vi "滾球機.vi"() -> ()   [LabVIEW 2018]
uses:
  <vilib>/myRIO/Common/Instrument Driver Framework/Utilities/typedefs/Generic FPGA Reference.ctl
  <vilib>/myRIO/Common/Instrument Driver Framework/Utilities/typedefs/myRIO v1.0 Reference.ctl
  <vilib>/myRIO/Common/Instrument Driver Framework/Utilities/typedefs/Hardware Version Enum.ctl
  <vilib>/myRIO/Common/Instrument Driver Framework/Utilities/typedefs/myRIO Generic Hardware Reference.ctl
  <vilib>/userdefined/High Color/nirio_resource_hc.ctl
  <vilib>/myRIO/Common/Instrument Driver Framework/Utilities/vis/Is FPGA Ref Available.vi
  <vilib>/myRIO/Express VI/Onboard IO/DI/DI Express VI.xnode
  <vilib>/myRIO/Instrument Drivers/Onboard IO/DIO/vis/Read.vi
  <vilib>/myRIO/Instrument Drivers/Onboard IO/DIO/DIO.lvlib
  <vilib>/myRIO/Common/Instrument Driver Framework/myRIO v1.0/DIO/typedefs/DIO Channels Enum.ctl
  <vilib>/myRIO/Common/Instrument Driver Framework/myRIO v1.0/DIO/typedefs/DIO Channels List.ctl
  <vilib>/myRIO/Instrument Drivers/Onboard IO/DIO/typedefs/DIO Reference.ctl
  <vilib>/myRIO/Instrument Drivers/Onboard IO/DIO/vis/myRIO DIO Open.xnode
  <vilib>/myRIO/Common/Instrument Driver Framework/myRIO v1.0/DIO/vis/myRIO v1.1 Open DIO.vi
  <vilib>/myRIO/Express VI/Onboard IO/PWM/PWM Express VI.xnode
  <vilib>/myRIO/Instrument Drivers/Onboard IO/PWM/vis/Set Duty Cycle and Frequency.vi
  <vilib>/myRIO/Instrument Drivers/Onboard IO/PWM/PWM.lvlib
  <vilib>/myRIO/Instrument Drivers/Onboard IO/PWM/typedefs/PWM Configuration.ctl
  <vilib>/myRIO/Common/Instrument Driver Framework/myRIO v1.0/PWM/typedefs/PWM Channels Enum.ctl
  <vilib>/myRIO/Instrument Drivers/Onboard IO/PWM/typedefs/PWM Reference.ctl
  <vilib>/myRIO/Instrument Drivers/Onboard IO/PWM/vis/myRIO PWM Open.xnode
  <vilib>/myRIO/Common/Instrument Driver Framework/myRIO v1.0/PWM/vis/myRIO v1.1 Open PWM.vi
panel:
  out "Tab Control":enum32{"Page 1", "Page 2"}(tab)
  in  "stop":bool
  in  "難度":bool
  out "String":string
  in  "OK Button 困難(雙人)":bool
  in  "OK Button 簡單(單人)":bool
  out "Boolean 5":bool
  out "Boolean 4":bool
  out "Boolean 3":bool
  out "Boolean 2":bool
  out "Boolean":bool
  in  "stop 2":bool
  out "得分":dbl
  out "總分":dbl
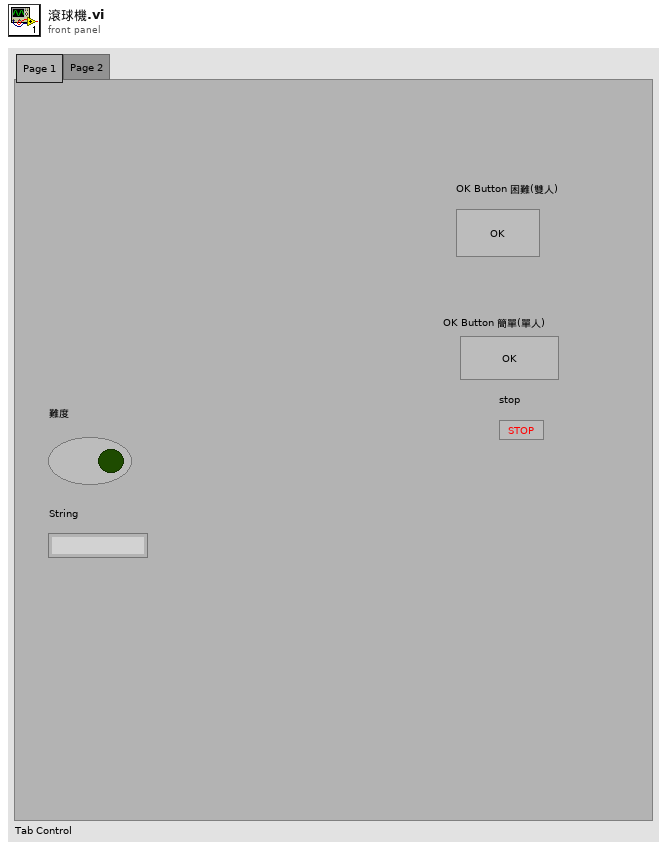
[diagram p1: front panel]
types:
  T1 = typedef "DIO.lvlib/DIO Reference.ctl" = cluster{"myRIO Reference":T2, "DIO Channels List":T6}
  T2 = typedef "myRIO Generic Hardware Reference.ctl" = cluster{"myRIO Model":T3, "myRIO Hardware Reference":T4}
  T3 = typedef "Hardware Version Enum.ctl" = enum16{"Unknown", "myRIO-1900", "myRIO-1950", "roboRIO", "NI ELVIS RIO CM", "ELVIS III"}
  T4 = typedef "myRIO v1.0 Reference.ctl" = cluster{"Generic FPGA Reference":T5, "Allow multiple opens":bool}
  T5 = typedef "Generic FPGA Reference.ctl" = refnum<k20>
  T6 = typedef "DIO Channels List.ctl" = T7[]
  T7 = typedef "DIO Channels Enum.ctl" = enum16{"Not Connected", "C/DIO0", "C/DIO1", "C/DIO2", "C/DIO3", "C/DIO4", "C/DIO5", "C/DIO6", "C/DIO7", "A/DIO0", "A/DIO1", "A/DIO2", "A/DIO3", "A/DIO4", "A/DIO5", "A/DIO6", "A/DIO7", "A/DIO8", "A/DIO9", "A/DIO10", "A/DIO11", "A/DIO12", "A/DIO13", "A/DIO14", "A/DIO15", "A/DIO16", "A/DIO17", "A/DIO18", "A/DIO19", "B/DIO0", "B/DIO1", "B/DIO2", "B/DIO3", "B/DIO4", "B/DIO5", "B/DIO6", "B/DIO7", "B/DIO8", "B/DIO9", "B/DIO10", "B/DIO11", "B/DIO12", "B/DIO13", "B/DIO14", "B/DIO15", "B/DIO16", "B/DIO17", "B/DIO18", "B/DIO19", "LED0", "LED1", "LED2", "LED3", "Button0", "DIO/DIO0", "DIO/DIO1", "DIO/DIO2", "DIO/DIO3", "DIO/DIO4", "DIO/DIO5", "DIO/DIO6", "DIO/DIO7", "DIO/DIO8", "DIO/DIO9", "SPI/CS0", "SPI/CS1", "SPI/CS2", "SPI/CS3", "LED RADIO (Green)", "LED RADIO (Red)", "LED COMM (Green)", "LED COMM (Red)", "LED MODE (Green)", "LED MODE (Red)"}
  T8 = typedef "nirio_resource_hc.ctl" = tag
  T9 = typedef "PWM.lvlib/PWM Reference.ctl" = cluster{"myRIO Reference":T2, "PWM Channels Enum":T10, "PWM Configuration":T11}
  T10 = typedef "PWM Channels Enum.ctl" = enum16{"Not Connected", "C/PWM0", "C/PWM1", "A/PWM0", "A/PWM1", "A/PWM2", "A/PWM3", "A/PWM4", "A/PWM5", "A/PWM6", "A/PWM7", "A/PWM8", "A/PWM9", "A/PWM10", "A/PWM11", "A/PWM12", "A/PWM13", "A/PWM14", "A/PWM15", "A/PWM16", "A/PWM17", "A/PWM18", "A/PWM19", "B/PWM0", "B/PWM1", "B/PWM2", "B/PWM3", "B/PWM4", "B/PWM5", "B/PWM6", "B/PWM7", "B/PWM8", "B/PWM9", "B/PWM10", "B/PWM11", "B/PWM12", "B/PWM13", "B/PWM14", "B/PWM15", "B/PWM16", "B/PWM17", "B/PWM18", "B/PWM19", "PWM/PWM0", "PWM/PWM1", "PWM/PWM2", "PWM/PWM3", "PWM/PWM4", "PWM/PWM5", "PWM/PWM6", "PWM/PWM7", "PWM/PWM8", "PWM/PWM9"}
  T11 = typedef "PWM.lvlib/PWM Configuration.ctl" = cluster{"Frequency":dbl, "Duty Cycle":dbl}
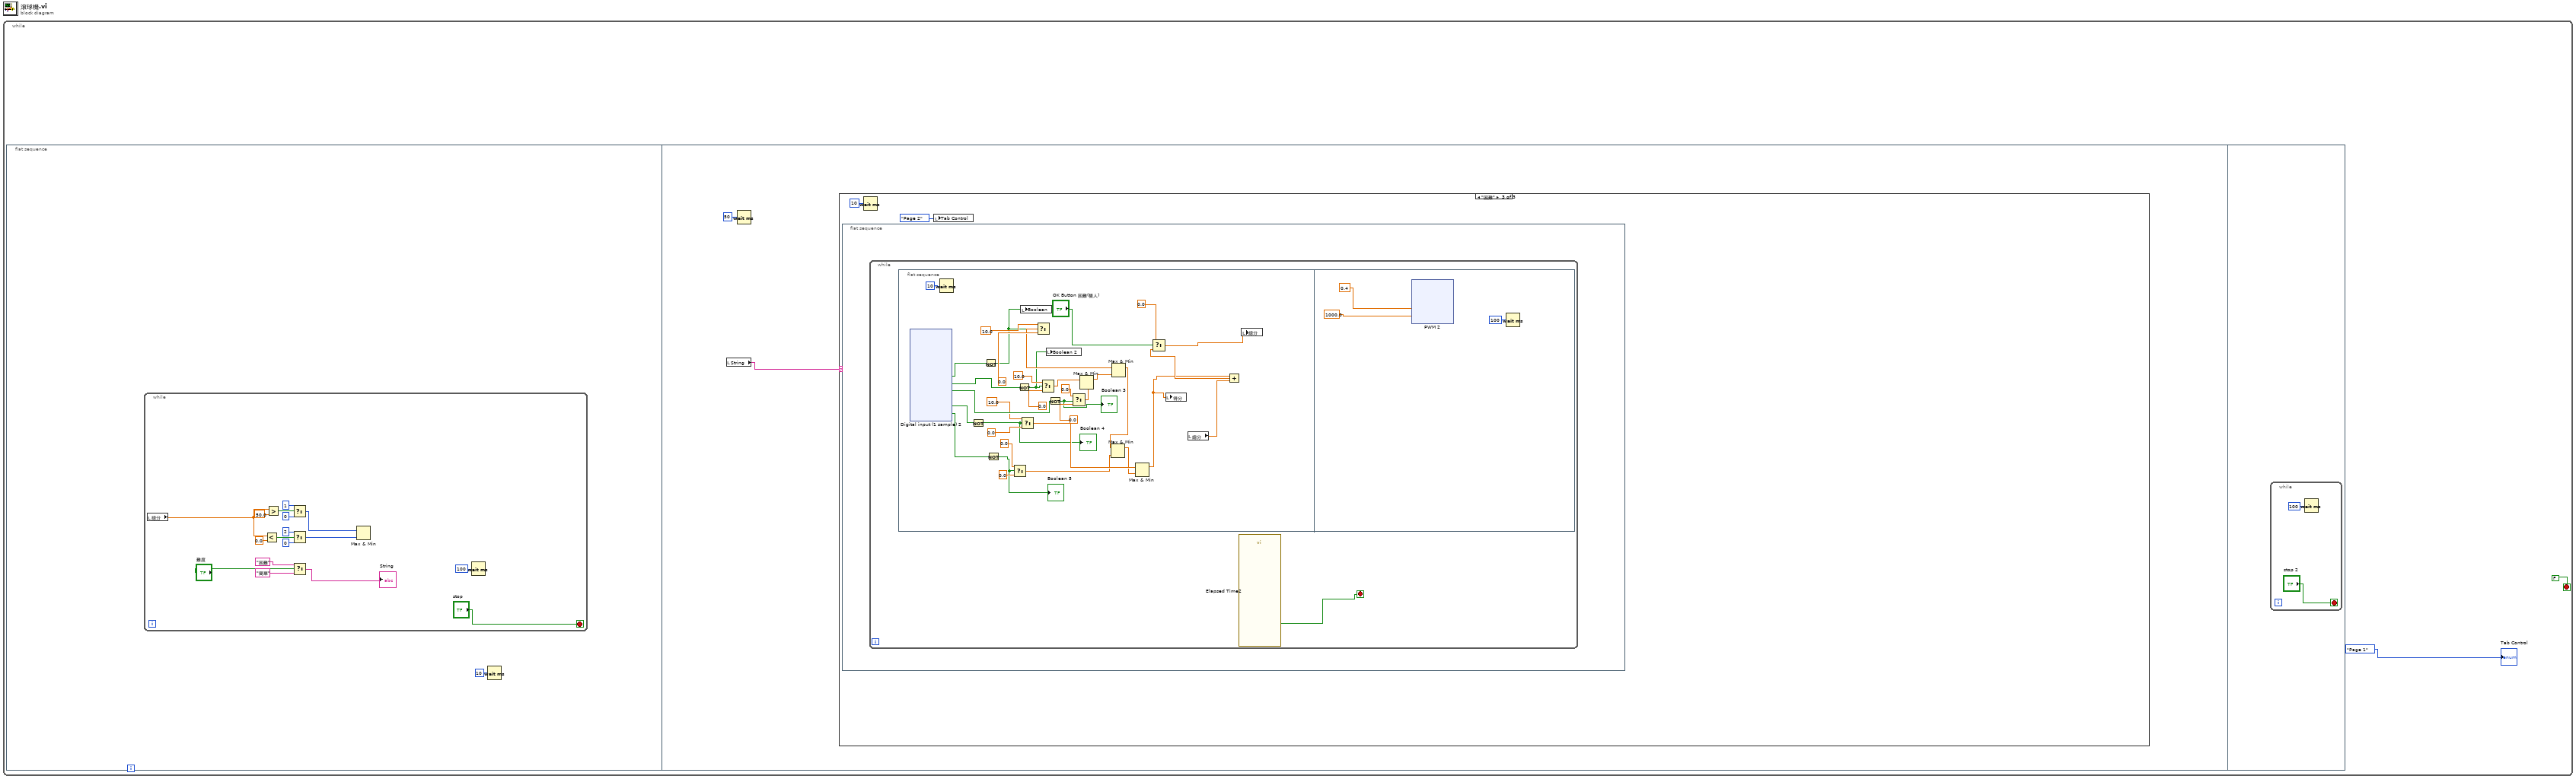
[diagram p0: block diagram]
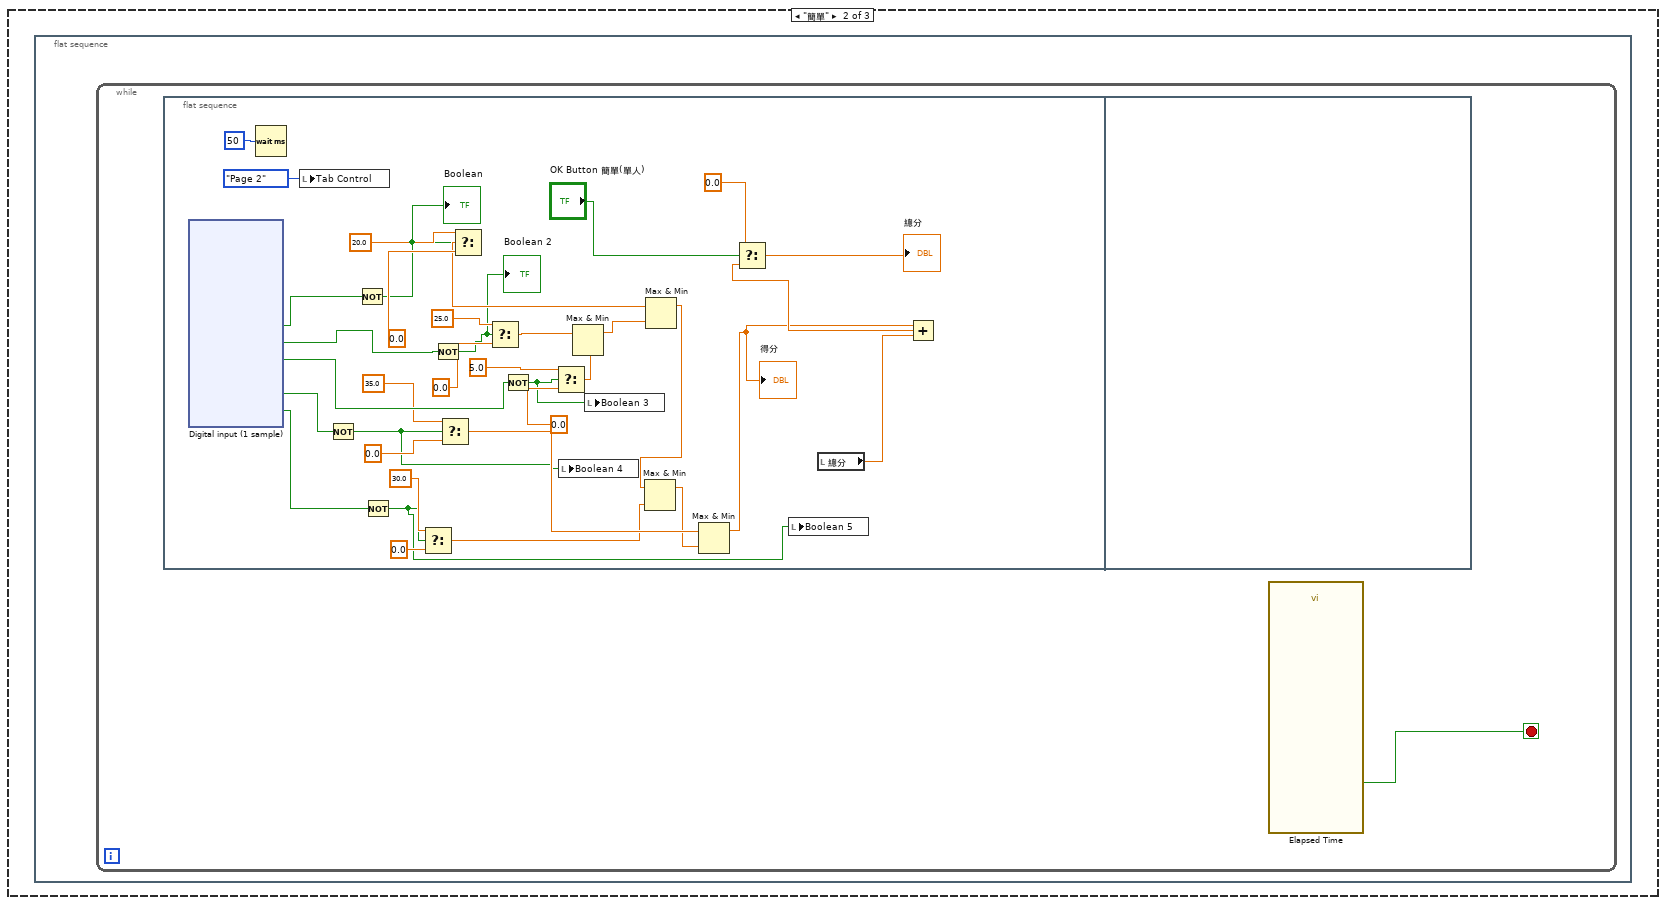
[diagram p3: hidden frame]
diagram:
  n1 = while {
    stop <- FALSE stop-if-true
    n2 = flat-sequence {
      frame #0 {
        n3 = while {
          stop <- "stop" stop-if-true
          n4 = local read "總分"() -> (w17:dbl)
          n5 = Less?(x=w17, y=0.0) -> (x < y?=w16:bool)
          n6 = Greater?(x=w17, y=50.0) -> (0:w18:bool)
          n7 = Select(t=u16 1, s=w18, f=u16 0) -> (s? t:f=w15:u16)
          n8 = Select(t=u16 2, s=w16, f=u16 0) -> (s? t:f=w14:u16)
          n9 = Select(t="困難" ("String"), s="難度", f="簡單" ("String")) -> (s? t:f=→"String":string)
          n10 = Max & Min(x=w15, y=w14) -> ()  [unwired: 2 out]
          n11 = Wait (ms)(milliseconds to wait=u32 100) -> ()  [unwired: 1 out]
        }
        n12 = Wait (ms)(milliseconds to wait=u32 10) -> ()  [unwired: 1 out]
      }
      frame #1 {
        n13 = local read "String"() -> (w22:string)
        n14 = Wait (ms)(milliseconds to wait=u32 50) -> ()  [unwired: 1 out]
        n15 = case shown="\"困難\"" w22 {
          frame "False", Default {
          }
          frame "簡單" {
            n16 = flat-sequence {
              frame #0 {
                n17 = while {
                  stop <- w23 stop-if-true
                  n18 = flat-sequence {
                    frame #0 {
                      n19 = xnode "Digital input (1 sample)"() -> ("A/DIO0 (Pin 11)"=w30:bool, "A/DIO1 (Pin 13)"=w52:bool, "A/DIO2 (Pin 15)"=w47:bool, "A/DIO3 (Pin 17)"=w39:bool, "A/DIO4 (Pin 19)"=w34:bool)  [unwired: 1 in, 2 out]
                      n20 = Wait (ms)(milliseconds to wait=u32 50) -> ()  [unwired: 1 out]
                      n21 = local write "Tab Control"(enum32{"Page 1", "Page 2"}."Page 2" ("Tab Control")) -> ()
                      n22 = Not(x=w39) -> (.not. x?=w25:bool)
                      n23 = Not(x=w30) -> (.not. x?=w28:bool)
                      "Boolean" <- w28
                      n24 = Not(x=w34) -> (.not. x?=w24:bool)
                      n25 = Select(t=30.0, s=w24, f=0.0) -> (s? t:f=w31:dbl)
                      n26 = Not(x=w52) -> (.not. x?=w27:bool)
                      "Boolean 2" <- w27
                      n27 = Select(t=35.0, s=w25, f=0.0) -> (s? t:f=w40:dbl)
                      n28 = Select(t=20.0, s=w28, f=0.0) -> (s? t:f=w56:dbl)
                      n29 = Select(t=25.0, s=w27, f=0.0) -> (s? t:f=w51:dbl)
                      n30 = Not(x=w47) -> (.not. x?=w26:bool)
                      n31 = Select(t=5.0, s=w26, f=0.0) -> (s? t:f=w41:dbl)
                      n32 = local write "Boolean 4"(w25) -> ()
                      n33 = Max & Min(x=w51, y=w41) -> (max(x,y)=w50:dbl)  [unwired: 1 out]
                      n34 = local write "Boolean 3"(w26) -> ()
                      n35 = Max & Min(x=w56, y=w50) -> (max(x,y)=w36:dbl)  [unwired: 1 out]
                      n36 = Max & Min(x=w36, y=w31) -> (max(x,y)=w35:dbl)  [unwired: 1 out]
                      n37 = Max & Min(x=w40, y=w35) -> (max(x,y)=w38:dbl)  [unwired: 1 out]
                      "得分" <- w38
                      n38 = local write "Boolean 5"(w24) -> ()
                      n39 = local read "總分"() -> (w37:dbl)
                      n40 = Add(x=w38, y=w37) -> (x+y=w46:dbl)
                      n41 = Select(t=0.0, s="OK Button 簡單(單人)", f=w46) -> (s? t:f=→"總分":dbl)
                    }
                    frame #1 {
                    }
                  }
                  n42 = call "Elapsed Time"() -> ("Time has Elapsed"=w23:bool)  [unwired: 12 in, 7 out]
                }
              }
            }
          }
          frame "困難" {
            n43 = flat-sequence {
              frame #0 {
                n44 = while {
                  stop <- w102 stop-if-true
                  n45 = flat-sequence {
                    frame #0 {
                      n46 = xnode "Digital input (1 sample) 2"() -> ("A/DIO0 (Pin 11)"=w111:bool, "A/DIO1 (Pin 13)"=w131:bool, "A/DIO2 (Pin 15)"=w126:bool, "A/DIO3 (Pin 17)"=w119:bool, "A/DIO4 (Pin 19)"=w115:bool)  [unwired: 1 in, 2 out]
                      n47 = Wait (ms)(milliseconds to wait=u32 10) -> ()  [unwired: 1 out]
                      n48 = Not(x=w119) -> (.not. x?=w104:bool)
                      "Boolean 4" <- w104
                      n49 = Not(x=w111) -> (.not. x?=w107:bool)
                      n50 = Not(x=w115) -> (.not. x?=w103:bool)
                      "Boolean 5" <- w103
                      n51 = Select(t=0.0, s=w103, f=0.0) -> (s? t:f=w112:dbl)
                      n52 = Not(x=w131) -> (.not. x?=w106:bool)
                      n53 = local write "Boolean"(w107) -> ()
                      n54 = Select(t=10.0, s=w104, f=0.0) -> (s? t:f=w120:dbl)
                      n55 = Select(t=10.0, s=w107, f=0.0) -> (s? t:f=w135:dbl)
                      n56 = Select(t=10.0, s=w106, f=0.0) -> (s? t:f=w130:dbl)
                      n57 = local write "Boolean 2"(w106) -> ()
                      n58 = Not(x=w126) -> (.not. x?=w105:bool)
                      "Boolean 3" <- w105
                      n59 = Select(t=0.0, s=w105, f=0.0) -> (s? t:f=w121:dbl)
                      n60 = Max & Min(x=w130, y=w121) -> (max(x,y)=w129:dbl)  [unwired: 1 out]
                      n61 = Max & Min(x=w135, y=w129) -> (max(x,y)=w117:dbl)  [unwired: 1 out]
                      n62 = Max & Min(x=w117, y=w112) -> (max(x,y)=w116:dbl)  [unwired: 1 out]
                      n63 = Max & Min(x=w120, y=w116) -> (max(x,y)=w109:dbl)  [unwired: 1 out]
                      n64 = local write "得分"(w109) -> ()
                      n65 = local read "總分"() -> (w118:dbl)
                      n66 = Add(x=w109, y=w118) -> (x+y=w125:dbl)
                      n67 = Select(t=0.0, s="OK Button 困難(雙人)", f=w125) -> (s? t:f=w110:dbl)
                      n68 = local write "總分"(w110) -> ()
                    }
                    frame #1 {
                      n69 = xnode "PWM 2"("Duty Cycle"=0.4, "Frequency [Hz]"=1000.0) -> ()  [unwired: 1 in, 1 out]
                      n70 = Wait (ms)(milliseconds to wait=u32 100) -> ()  [unwired: 1 out]
                    }
                  }
                  n71 = call "Elapsed Time2"() -> ("Time has Elapsed"=w102:bool)  [unwired: 12 in, 7 out]
                }
              }
            }
            n72 = Wait (ms)(milliseconds to wait=u32 10) -> ()  [unwired: 1 out]
            n73 = local write "Tab Control"(enum32{"Page 1", "Page 2"}."Page 2" ("Tab Control")) -> ()
          }
        }
      }
      frame #2 {
        n74 = while {
          stop <- "stop 2" stop-if-true
          n75 = Wait (ms)(milliseconds to wait=u32 100) -> ()  [unwired: 1 out]
        }
      }
    }
    "Tab Control" <- enum32{"Page 1", "Page 2"}."Page 1" ("Tab Control")
  }
